vi "Unit Test launcher.vi"() -> ()   [LabVIEW 2020]
uses:
  Unit_Test_NI6008.lvclass
  C:/Program Files/National Instruments/LabVIEW 2020/vi.lib/ActorFramework/Actor/Actor.lvclass
  <vilib>/ActorFramework/Actor/Actor.lvclass
panel:
  in  "Choose NI 6008 Resource":tag="Dev1"
  in  "stop":bool
  out "NI6008 Tester Active":bool
  in  "NI6008 Tester":bool
  # "Pulse Gen Unit Test Panel"
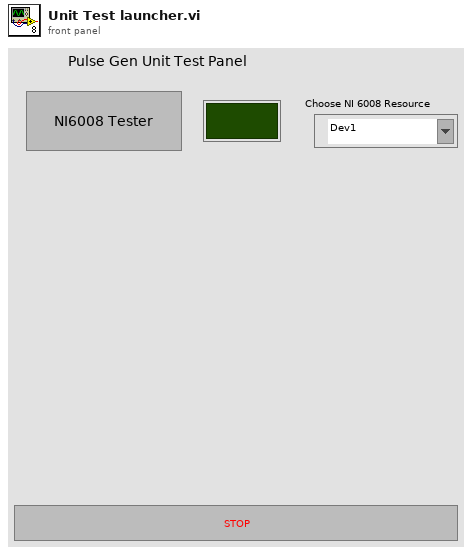
[diagram p1: front panel]
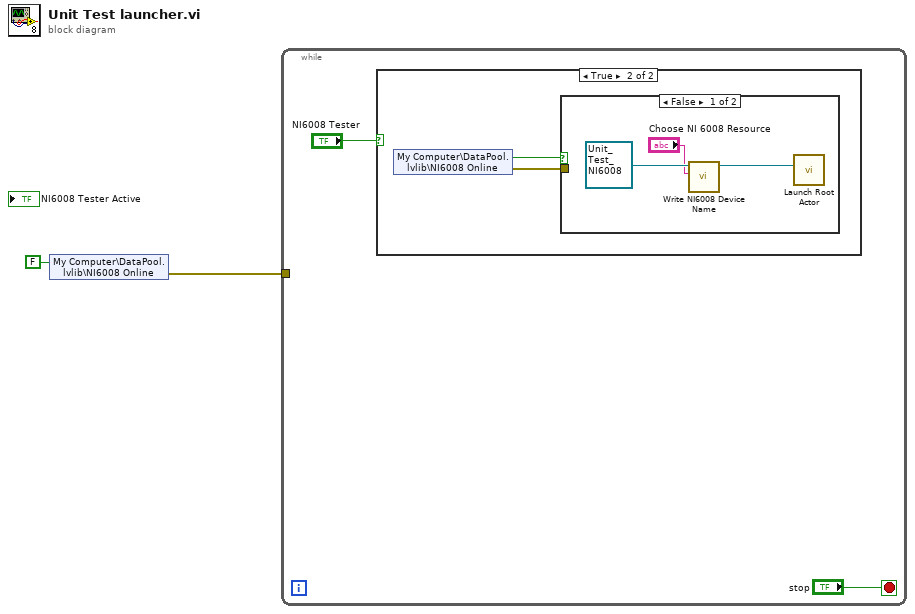
[diagram p0: block diagram]
diagram:
  n1 = shared-variable "My Computer\\DataPool.lvlib\\NI6008 Online"(FALSE ("NI6008 Tester Active")) -> (error out=w1:errorcluster)  [unwired: 1 in]
  n2 = while {
    tunnel: w1 -> [_]
    stop <- "stop" stop-if-true
    n3 = case shown="True" "NI6008 Tester" {
      frame False {
      }
      frame True {
        n4 = shared-variable "My Computer\\DataPool.lvlib\\NI6008 Online"() -> (w6:bool, error out=w5:errorcluster)  [unwired: 1 in]
        n5 = case shown="False" w6 {
          tunnel: w5 -> [_ _]
          frame False {
            n6 = call-dynamic "Write NI6008 Device Name.vi"("NI6008 Device Name"="Choose NI 6008 Resource", "Unit_Test_NI6008 in"=refnum<class "Unit_Test_NI6008.lvclass"> refnum ("Unit_Test_NI6008.lvlib:Unit_Test_NI6008.lvclass")) -> ("Unit_Test_NI6008 out"=w8:refnum<class "Unit_Test_NI6008.lvclass">)  [unwired: 8 in, 1 out]
            n7 = call <vilib>:"Launch Root Actor.vi"("Actor"=w8) -> ()  [unwired: 9 in, 2 out]
          }
          frame True {
          }
        }
      }
    }
  }
